vi "Open.vi"(8 "error in (no error)":errorcluster, 11 "Axis":refnum<k21>) -> (0 "error out":errorcluster, 3 "Base Axis Out":refnum<class "nismPluginAxisBaseClass.lvclass">)   [LabVIEW 2014, in "Template SoftMotion Drive Interface Plug-in Class.lvclass"]
uses:
  Template SoftMotion Drive Interface Plug-in Class.lvclass
  <vilib>/Motion/plugins/PluginFramework/nismPluginAxisBase/nismPluginAxisBaseClass.lvclass
  <vilib>/Motion/plugins/PluginFramework/nismPluginAxisBase/nismPluginAxisBaseClass.lvclass/nismPluginAxisBaseClass.ctl
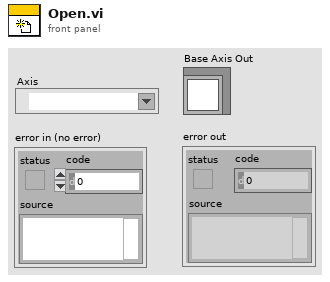
[diagram p1: front panel]
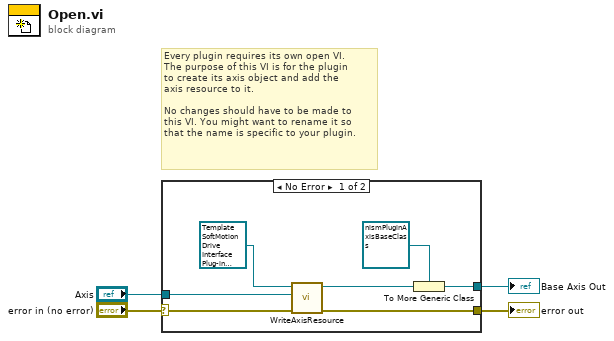
[diagram p0: block diagram]
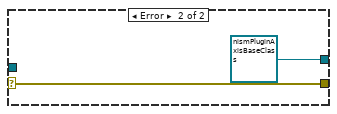
[diagram p2: hidden frame]
diagram:
  # "Every plugin requires its own open VI.\nThe purpose of this VI is for the plugin\nto create its axis object and add the \naxis resource to it.\n\nNo changes should have to be made to\nthis VI. You might want to rename it so \nthat the name is specific to your plugin."
  n1 = case shown="No Error" "error in (no error)" {
    selector: "error in (no error)" -> [w7 w13]
    tunnel: [w5 w13] -> w3
    tunnel: [w6 refnum<class "nismPluginAxisBaseClass.lvclass"> refnum ("nismPluginAxisBaseClass.lvclass")] -> w1
    tunnel: "Axis" -> [w8 _]
    frame No Error {
      n2 = call <vilib>:"WriteAxisResource.vi"("error in (no error)"=w7, "Axis Resource"=w8, "nismPluginAxisBaseClass in"=refnum<class "Template SoftMotion Drive Interface Plug-in Class.lvclass"> refnum ("Template Plugin Class.lvclass")) -> ("error out"=w5:errorcluster, "nismPluginAxisBaseClass out"=w11:refnum<class "Template SoftMotion Drive Interface Plug-in Class.lvclass">)  [unwired: 7 in]
      n3 = To More Generic Class(target class=refnum<class "nismPluginAxisBaseClass.lvclass"> refnum ("nismPluginAxisBaseClass.lvclass"), reference=w11) -> (generic class reference=w6:refnum<class "nismPluginAxisBaseClass.lvclass">)
    }
    frame Error {
    }
  }
  "error out" <- w3
  "Base Axis Out" <- w1
